vi "write_parameters_csv_from_calibration.vi"(8 "error in (no error)":errorcluster, 10 "parameter, value pairs":string[][](array[string]), 11 "Computer Name":string) -> (0 "error out":errorcluster)   [LabVIEW 2019]
uses:
  <vilib>/Utility/file.llb/Read Delimited Spreadsheet (string).vi
  <vilib>/Utility/file.llb/Write Delimited Spreadsheet (string).vi
panel:
  out "rewritten csv":string[][](array[string])
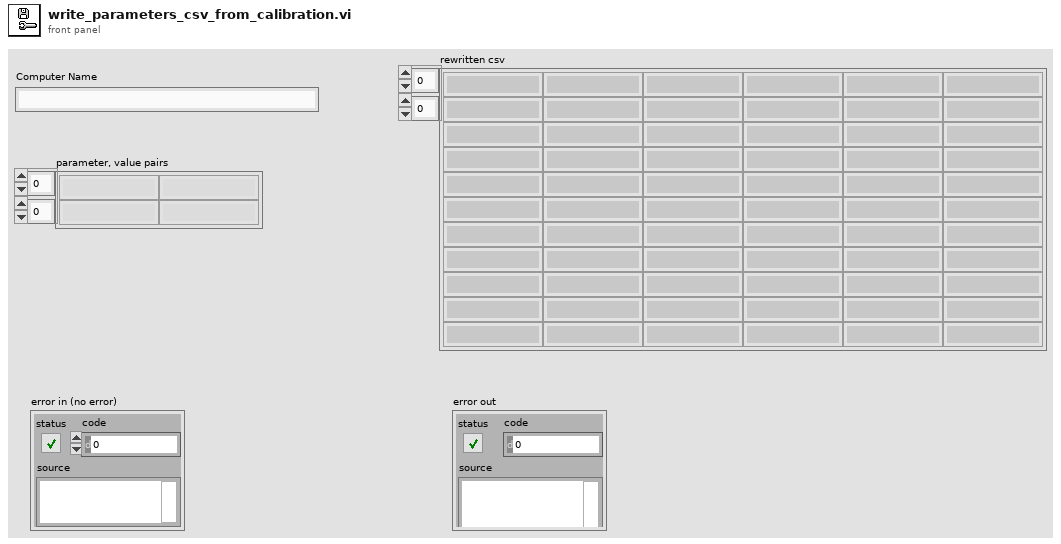
[diagram p1: front panel]
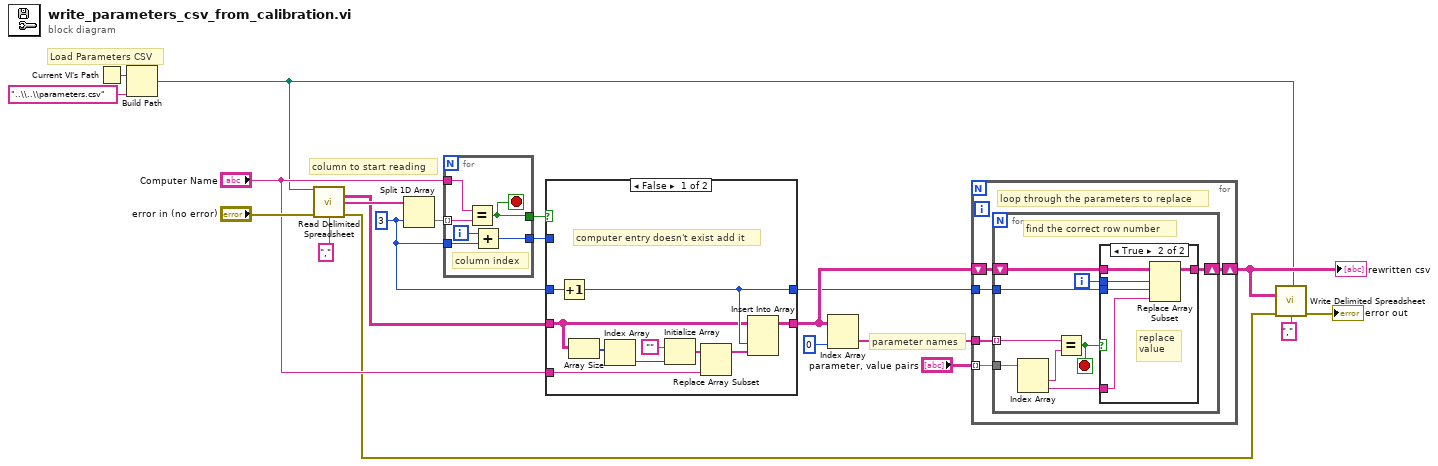
[diagram p0: block diagram]
diagram:
  w9 = 3 ("y")
  # "parameter names"
  # "column to start reading"
  # "Load Parameters CSV"
  n1 = Current VI's Path() -> (path=w15:path)
  n2 = Build Path(base path=w15, name or relative path="..\\..\\parameters.csv") -> (appended path=w3:path)
  n3 = call-poly <vilib>:"Read Delimited Spreadsheet.vi"("file path (dialog if empty)"=w3, "error in (no error)"="error in (no error)", "delimiter (\\t)"=",") -> ("all rows"=w11:string[][], "first row"=w17:string[], "error out"=w1:errorcluster)  [unwired: 7 in, 3 out]
  n4 = Split 1D Array(array=w17, index=w9) -> (second subarray=w16:string[])  [unwired: 1 out]
  n5 = for {
    tunnel: "Computer Name" -> [w24]
    tunnel: w16 -> [w25] mode=indexing
    tunnel: w9 -> [w26]
    tunnel: [w23] -> w12
    tunnel: [w22] -> w10
    i -> [w27]
    stop <- w23 stop-if-true
    # "column index"
    n6 = Equal?(x=w24, y=w25) -> (x = y?=w23:bool)
    n7 = Add(x=w27, y=w26) -> (x+y=w22:i32)
  }
  n8 = case shown="False" w12 {
    tunnel: w11 -> [w30 w38]
    tunnel: [w36 w39] -> w6
    tunnel: w10 -> [_ w39]
    tunnel: [w37 w38] -> w7
    tunnel: w9 -> [w35 _]
    tunnel: "Computer Name" -> [w32 _]
    frame False {
      # "computer entry doesn't exist add it"
      n9 = Increment(x=w35) -> (x+1=w36:i32)
      n10 = Array Size(array=w30) -> (size(s)=w29:i32[])
      n11 = Index Array(array=w29) -> (element=w28:i32)  [unwired: 1 in]
      n12 = Initialize Array("", w28) -> (w33:string[])
      n13 = Replace Array Subset(array=w33, new element=w32) -> (w31:string[])  [unwired: 1 in]
      n14 = Insert Into Array(array=w30, index (col)=w36, new element=w31) -> (w37:string[][])  [unwired: 1 in]
    }
    frame True {
      # "computer entry exists,\nreplace existing entries"
    }
  }
  n15 = Index Array(array=w7, index (col)=0) -> (element=w8:string[])  [unwired: 1 in]
  n16 = for {
    tunnel: "parameter, value pairs" -> [w43] mode=indexing
    tunnel: w8 -> [w44]
    shift-right: [w41] -> w5
    shift-left: w7 -> [w42]
    tunnel: w6 -> [w40]
    # "loop through the parameters to replace"
    n17 = for {
      tunnel: w44 -> [w52] mode=indexing
      tunnel: w43 -> [w53]
      shift-right: [w47] -> w41
      shift-left: w42 -> [w48]
      tunnel: w40 -> [w46]
      i -> [w45]
      stop <- w50 stop-if-true
      # "find the correct row number"
      n18 = Index Array(array=w53) -> (element #1=w51:string, element #2=w49:string)  [unwired: 2 in]
      n19 = Equal?(x=w52, y=w51) -> (x = y?=w50:bool)
      n20 = case shown="True" w50 {
        tunnel: w49 -> [_ w55]
        tunnel: w48 -> [w54 w59]
        tunnel: [w54 w58] -> w47
        tunnel: w46 -> [_ w56]
        tunnel: w45 -> [_ w57]
        frame False {
        }
        frame True {
          # "replace \nvalue"
          n21 = Replace Array Subset(array=w59, new element=w55, index (row)=w57, index (col)=w56) -> (w58:string[][])
        }
      }
    }
  }
  "rewritten csv" <- w5
  n22 = call-poly <vilib>:"Write Delimited Spreadsheet.vi"("file path (dialog if empty)"=w3, "2D data"=w5, "error in (no error)"=w1, "delimiter (\\t)"="," ("delimiter (\\t)")) -> ("error out"=→"error out":errorcluster)  [unwired: 10 in, 1 out]
